vi "Add Performance Channel to All Plugins.vi"(7 "GUID (Default Channel)":string="03D3BB99-1485-13A6-561D1F898F032919", 8 "error in (no error)":errorcluster, 9 "Channel":T1, 10 "Channel Name":string, 11 "Item Ref in":T3 format="%.0x") -> (0 "error out":errorcluster, 3 "Item Ref out":T3 format="%.0x")   [LabVIEW 2017]
uses:
  <vilib>/NI Veristand/Custom Device API/Custom Device Item Ref.ctl
  <vilib>/NI Veristand/Custom Device API/Custom Device Channel.ctl
  <vilib>/NI Veristand/Custom Device API/Custom Device Channel Type.ctl
  <vilib>/NI Veristand/Custom Device API/Custom Device API.lvlib
  Shared/DSF Shared.lvlib
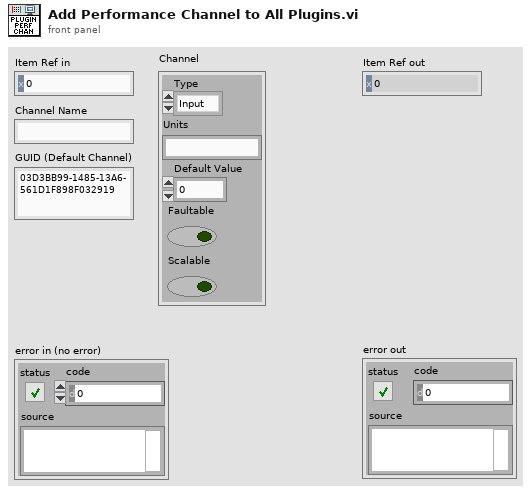
[diagram p1: front panel]
types:
  T1 = typedef "Custom Device API.lvlib/Custom Device Channel.ctl" = cluster{"Type":T2, "Units":string, "Default Value":dbl, "Faultable":bool, "Scalable":bool}
  T2 = typedef "Custom Device API.lvlib/Custom Device Channel Type.ctl" = enum16{"Input", "Output"}
  T3 = typedef "Custom Device API.lvlib/Custom Device Item Ref.ctl" = u64
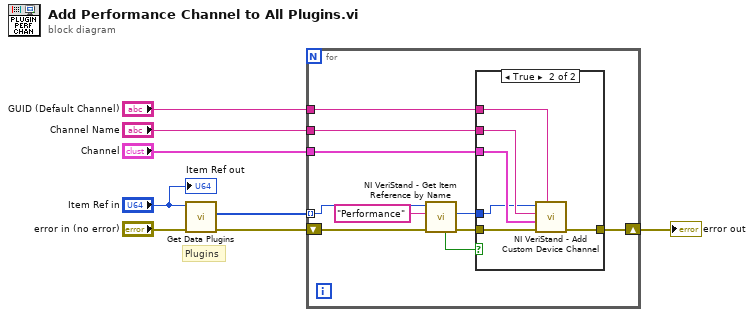
[diagram p0: block diagram]
diagram:
  # "Plugins"
  n1 = call "Get Data Plugins.vi"("error in (no error)"="error in (no error)", "Framework Ref in"="Item Ref in") -> ("error out"=w3:errorcluster, "Plugin refs"=w2:T3[])  [unwired: 7 in, 1 out]
  n2 = for {
    shift-right: [w10] -> w8
    shift-left: w3 -> [w14]
    tunnel: w2 -> [w11] mode=indexing
    tunnel: "Channel Name" -> [w13]
    tunnel: "Channel" -> [w9]
    tunnel: "GUID (Default Channel)" -> [w12]
    n3 = call <vilib>:"NI VeriStand - Get Item Reference by Name.vi"("error in (no error)"=w14, "Item Name"="Performance", "Parent Ref in"=w11) -> ("error out"=w16:errorcluster, "Item Ref"=w15:T3, "Found"=w17:bool)  [unwired: 5 in, 1 out]
    n4 = case shown="True" w17 {
      tunnel: w16 -> [w19 w25]
      tunnel: w15 -> [_ w21]
      tunnel: [w19 w20] -> w10
      tunnel: w9 -> [_ w24]
      tunnel: w13 -> [_ w23]
      tunnel: w12 -> [_ w22]
      frame False {
      }
      frame True {
        n5 = call <vilib>:"NI VeriStand - Add Custom Device Channel.vi"("GUID (Default Channel)"=w22, "error in (no error)"=w25, "Channel"=w24, "Channel Name"=w23, "Parent Ref in"=w21) -> ("error out"=w20:errorcluster)  [unwired: 3 in, 3 out]
      }
    }
  }
  "error out" <- w8
  "Item Ref out" <- "Item Ref in"
